vi "EXO3.vi"() -> ()   [LabVIEW 2019]
uses:
  <vilib>/myRIO/Instrument Drivers/Onboard Devices/Accelerometer/typedefs/Accelerometer Reference.ctl
  <vilib>/myRIO/Common/Instrument Driver Framework/Utilities/typedefs/myRIO Generic Hardware Reference.ctl
  <vilib>/myRIO/Common/Instrument Driver Framework/Utilities/typedefs/Hardware Version Enum.ctl
  <vilib>/myRIO/Common/Instrument Driver Framework/Utilities/typedefs/myRIO v1.0 Reference.ctl
  <vilib>/myRIO/Common/Instrument Driver Framework/Utilities/typedefs/Generic FPGA Reference.ctl
  <vilib>/myRIO/Common/Instrument Driver Framework/myRIO v1.0/Accelerometer/typedefs/Accelerometer Channels List.ctl
  <vilib>/myRIO/Common/Instrument Driver Framework/myRIO v1.0/Accelerometer/typedefs/Accelerometer Channels Enum.ctl
  <vilib>/userDefined/High Color/nirio_resource_hc.ctl
  <vilib>/myRIO/Instrument Drivers/Onboard IO/DIO/typedefs/DIO Reference.ctl
  <vilib>/myRIO/Common/Instrument Driver Framework/myRIO v1.0/DIO/typedefs/DIO Channels List.ctl
  <vilib>/myRIO/Common/Instrument Driver Framework/myRIO v1.0/DIO/typedefs/DIO Channels Enum.ctl
  <vilib>/myRIO/Common/Instrument Driver Framework/Utilities/vis/Is FPGA Ref Available.vi
  <vilib>/myRIO/Common/Instrument Driver Framework/myRIO v1.0/Accelerometer/vis/myRIO v1.1 Open Accelerometer.vi
  <vilib>/myRIO/Instrument Drivers/Onboard Devices/Accelerometer/vis/Read.vi
  <vilib>/myRIO/Common/Instrument Driver Framework/myRIO v1.0/DIO/vis/myRIO v1.1 Open DIO.vi
  <vilib>/myRIO/Instrument Drivers/Onboard IO/DIO/vis/Write.vi
  <vilib>/myRIO/Common/Instrument Driver Framework/Utilities/vis/Validate Channels.vi
  <vilib>/myRIO/Common/Instrument Driver Framework/myRIO v1.0/Accelerometer/vis/myRIO v1.0 Reserve Accelerometer.vi
  <vilib>/myRIO/Common/Instrument Driver Framework/myRIO v1.0/DIO/vis/myRIO v1.0 Reserve DIO.vi
  <vilib>/myRIO/Common/Instrument Driver Framework/myRIO v1.0/Resource Manager/vis/myRIO v1.0 Reserve Channel List.vi
  <vilib>/myRIO/Common/Instrument Driver Framework/myRIO v1.0/Accelerometer/vis/myRIO v1.0 Build MUX Configuration Accelerometer.vi
  <vilib>/myRIO/Common/Instrument Driver Framework/myRIO v1.0/DIO/vis/myRIO v1.0 Build MUX Configuration DIO.vi
  <vilib>/myRIO/Common/Instrument Driver Framework/myRIO v1.0/Resource Manager/vis/myRIO v1.0 Reserve Channel.vi
  <vilib>/myRIO/Common/Instrument Driver Framework/myRIO v1.0/Resource Manager/vis/myRIO v1.0 Unreserve Channel.vi
  <vilib>/myRIO/Common/Instrument Driver Framework/myRIO v1.0/Resource Manager/vis/myRIO v1.0 Create Configuration List.vi
  <vilib>/myRIO/Common/Instrument Driver Framework/myRIO v1.0/Resource Manager/vis/myRIO v1.0 Build Mutex Name.vi
  <vilib>/Utility/VariantDataType/GetNumericInfo.vi
  <vilib>/Utility/error.llb/Error Cluster From Error Code.vi
  <vilib>/myRIO/Common/Instrument Driver Framework/myRIO v1.0/myRIO v1.1 Open.vi
  <vilib>/myRIO/Common/Instrument Driver Framework/myRIO v1.0/Accelerometer/vis/myRIO v1.0 Get Scaling Constant Accelerometer.vi
  <vilib>/myRIO/Common/Instrument Driver Framework/Utilities/vis/IO Manager.vi
  <vilib>/myRIO/Common/Instrument Driver Framework/Utilities/vis/Configuration Manager.vi
  <vilib>/myRIO/Common/Instrument Driver Framework/myRIO v1.0/myRIO v1.0 Close.vi
  <vilib>/myRIO/Common/Instrument Driver Framework/myRIO v1.0/Accelerometer/vis/myRIO v1.0 Read Accelerometer.vi
  <vilib>/myRIO/Common/Instrument Driver Framework/myRIO v1.0/Resource Manager/vis/myRIO v1.0 Configure IO.vi
  <vilib>/myRIO/Common/Instrument Driver Framework/myRIO v1.0/DIO/vis/myRIO v1.0 Write DIO.vi
  <vilib>/myRIO/Express VI/Onboard Devices/Accelerometer/Accelerometer Express VI.xnode
  <vilib>/myRIO/Instrument Drivers/Onboard Devices/Accelerometer/vis/myRIO Accelerometer Open.xnode
  <vilib>/myRIO/Express VI/Onboard Devices/LED/LED Express VI.xnode
  <vilib>/myRIO/Instrument Drivers/Onboard IO/DIO/vis/myRIO DIO Open.xnode
  <vilib>/myRIO/Instrument Drivers/Onboard Devices/Accelerometer/Accelerometer.lvlib
  <vilib>/myRIO/Instrument Drivers/Onboard IO/DIO/DIO.lvlib
panel:
  in  "?":bool
  out "Inclinaison en degré":dbl
  out "Z":dbl
  out "Y":dbl
  out "X":dbl
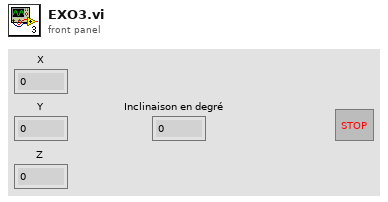
[diagram p1: front panel]
types:
  T1 = typedef "DIO.lvlib/DIO Reference.ctl" = cluster{"myRIO Reference":T2, "DIO Channels List":T6}
  T2 = typedef "myRIO Generic Hardware Reference.ctl" = cluster{"myRIO Model":T3, "myRIO Hardware Reference":T4}
  T3 = typedef "Hardware Version Enum.ctl" = enum16{"Unknown", "myRIO-1900", "myRIO-1950", "roboRIO", "NI ELVIS RIO CM", "ELVIS III"}
  T4 = typedef "myRIO v1.0 Reference.ctl" = cluster{"Generic FPGA Reference":T5, "Allow multiple opens":bool}
  T5 = typedef "Generic FPGA Reference.ctl" = refnum<k20>
  T6 = typedef "DIO Channels List.ctl" = T7[]
  T7 = typedef "DIO Channels Enum.ctl" = enum16{"Not Connected", "C/DIO0", "C/DIO1", "C/DIO2", "C/DIO3", "C/DIO4", "C/DIO5", "C/DIO6", "C/DIO7", "A/DIO0", "A/DIO1", "A/DIO2", "A/DIO3", "A/DIO4", "A/DIO5", "A/DIO6", "A/DIO7", "A/DIO8", "A/DIO9", "A/DIO10", "A/DIO11", "A/DIO12", "A/DIO13", "A/DIO14", "A/DIO15", "A/DIO16", "A/DIO17", "A/DIO18", "A/DIO19", "B/DIO0", "B/DIO1", "B/DIO2", "B/DIO3", "B/DIO4", "B/DIO5", "B/DIO6", "B/DIO7", "B/DIO8", "B/DIO9", "B/DIO10", "B/DIO11", "B/DIO12", "B/DIO13", "B/DIO14", "B/DIO15", "B/DIO16", "B/DIO17", "B/DIO18", "B/DIO19", "LED0", "LED1", "LED2", "LED3", "Button0", "DIO/DIO0", "DIO/DIO1", "DIO/DIO2", "DIO/DIO3", "DIO/DIO4", "DIO/DIO5", "DIO/DIO6", "DIO/DIO7", "DIO/DIO8", "DIO/DIO9", "SPI/CS0", "SPI/CS1", "SPI/CS2", "SPI/CS3", "LED RADIO (Green)", "LED RADIO (Red)", "LED COMM (Green)", "LED COMM (Red)", "LED MODE (Green)", "LED MODE (Red)"}
  T8 = typedef "nirio_resource_hc.ctl" = tag
  T9 = typedef "Accelerometer.lvlib/Accelerometer Reference.ctl" = cluster{"myRIO Reference":T2, "Accelerometer Channels List":T10, "LSB Weight":dbl}
  T10 = typedef "Accelerometer Channels List.ctl" = T11[]
  T11 = typedef "Accelerometer Channels Enum.ctl" = enum16{"Not Connected", "X-Axis", "Y-Axis", "Z-Axis"}
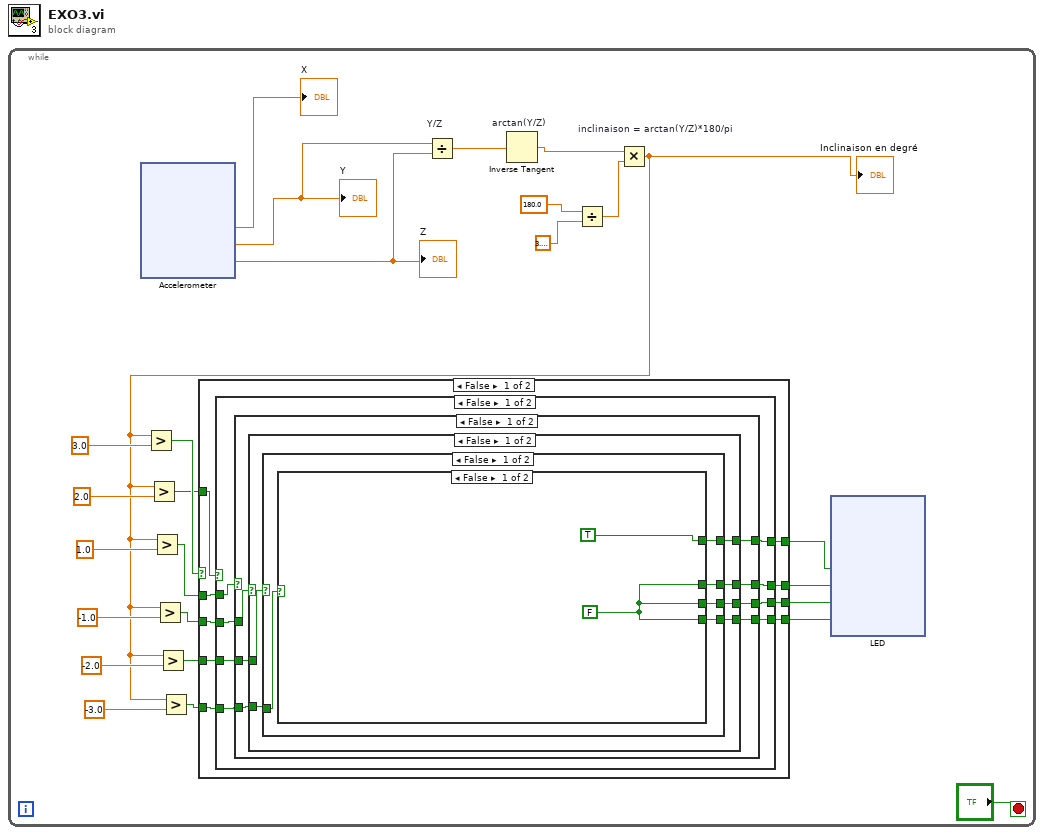
[diagram p0: block diagram]
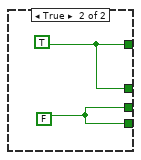
[diagram p2: hidden frame]
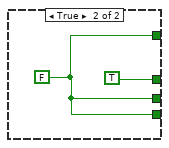
[diagram p3: hidden frame]
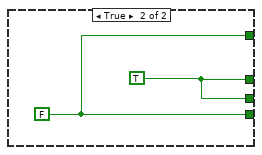
[diagram p4: hidden frame]
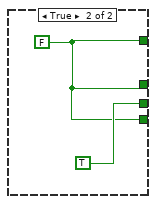
[diagram p5: hidden frame]
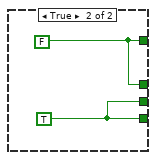
[diagram p6: hidden frame]
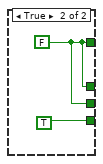
[diagram p7: hidden frame]
diagram:
  n1 = while {
    stop <- "?" stop-if-true
    n2 = xnode "Accelerometer"() -> ("X"=→"X":dbl, "Y"=w25:dbl, "Z"=w24:dbl)  [unwired: 1 in, 1 out]
    "Y" <- w25
    "Z" <- w24
    n3 = Divide "Y/Z"(x=w25, y=w24) -> (x/y=w23:dbl)
    n4 = Inverse Tangent "arctan(Y/Z)"(1:w23) -> (0:w20:dbl)
    n5 = Divide(x=180.0, y=3.141592653589793) -> (x/y=w19:dbl)
    n6 = Multiply "inclinaison = arctan(Y/Z)*180/pi"(x=w20, y=w19) -> (x*y=w1:dbl)
    "Inclinaison en degré" <- w1
    n7 = Greater?(x=w1, y=3.0) -> (0:w11:bool)
    n8 = Greater?(x=w1, y=2.0) -> (0:w10:bool)
    n9 = Greater?(x=w1, y=1.0) -> (0:w9:bool)
    n10 = Greater?(x=w1, y=-1.0) -> (0:w7:bool)
    n11 = Greater?(x=w1, y=-2.0) -> (0:w5:bool)
    n12 = Greater?(x=w1, y=-3.0) -> (0:w3:bool)
    n13 = case shown="False" w11 {
      tunnel: [w33 w75] -> w18
      tunnel: [w32 w75] -> w17
      tunnel: [w34 w75] -> w16
      tunnel: [w35 TRUE] -> w15
      tunnel: w10 -> [w31 _]
      tunnel: w9 -> [w30 _]
      tunnel: w7 -> [w29 _]
      tunnel: w5 -> [w28 _]
      tunnel: w3 -> [w27 _]
      frame False {
        n14 = case shown="False" w31 {
          tunnel: [w40 w73] -> w35
          tunnel: [w43 w73] -> w34
          tunnel: [w42 w72] -> w33
          tunnel: [w41 w72] -> w32
          tunnel: w30 -> [w39 _]
          tunnel: w29 -> [w38 _]
          tunnel: w28 -> [w37 _]
          tunnel: w27 -> [w36 _]
          frame False {
            n15 = case shown="False" w39 {
              tunnel: [w48 TRUE] -> w43
              tunnel: [w47 w70] -> w42
              tunnel: [w49 w70] -> w41
              tunnel: [w46 w70] -> w40
              tunnel: w38 -> [w50 _]
              tunnel: w37 -> [w45 _]
              tunnel: w36 -> [w44 _]
              frame False {
                n16 = case shown="False" w50 {
                  tunnel: [w55 w69] -> w49
                  tunnel: [w52 w69] -> w48
                  tunnel: [w54 w68] -> w47
                  tunnel: [w53 w68] -> w46
                  tunnel: w45 -> [w56 _]
                  tunnel: w44 -> [w51 _]
                  frame False {
                    n17 = case shown="False" w56 {
                      tunnel: [w59 TRUE] -> w55
                      tunnel: [w60 w66] -> w54
                      tunnel: [w57 w66] -> w53
                      tunnel: [w58 w66] -> w52
                      tunnel: w51 -> [w61 _]
                      frame False {
                        n18 = case shown="False" w61 {
                          tunnel: [TRUE w65] -> w60
                          tunnel: [w62 w65] -> w59
                          tunnel: [w62 w64] -> w58
                          tunnel: [w62 w64] -> w57
                          frame False {
                            w62 = FALSE
                          }
                          frame True {
                            w65 = TRUE
                            w64 = FALSE
                          }
                        }
                      }
                      frame True {
                        w66 = FALSE
                      }
                    }
                  }
                  frame True {
                    w69 = TRUE
                    w68 = FALSE
                  }
                }
              }
              frame True {
                w70 = FALSE
              }
            }
          }
          frame True {
            w72 = FALSE
            w73 = TRUE
          }
        }
      }
      frame True {
        w75 = FALSE
      }
    }
    n19 = xnode "LED"("LED0"=w18, "LED1"=w17, "LED2"=w16, "LED3"=w15) -> ()  [unwired: 1 in, 1 out]
  }
